vi "SetXAxisFormat.vi"(1 "Waveform Chart Reference":refnum<vi>) -> ()   [LabVIEW 2019]
uses:
  <vilib>/Utility/config.llb/Read Key (String).vi
  <vilib>/Utility/config.llb/NI_LVConfig.lvlib
panel:
  in  "Error In":errorcluster
  out "Error Out":errorcluster
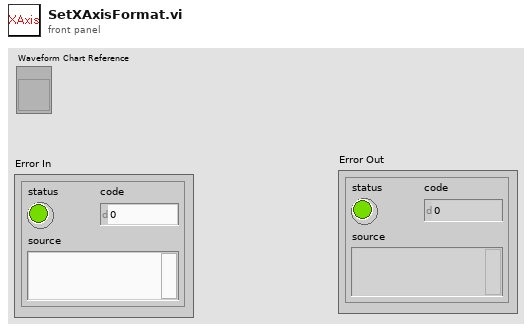
[diagram p1: front panel]
types:
  T1 = cluster{"XScale.Format":u8, "XScale.FormatString":string}[]
  T2 = typedef "NI_LVConfig.lvlib/Config Data RefNum.ctl" = refnum<k1>
  T3 = cluster{"XScale.Format":u8, "XScale.FormatString":string}
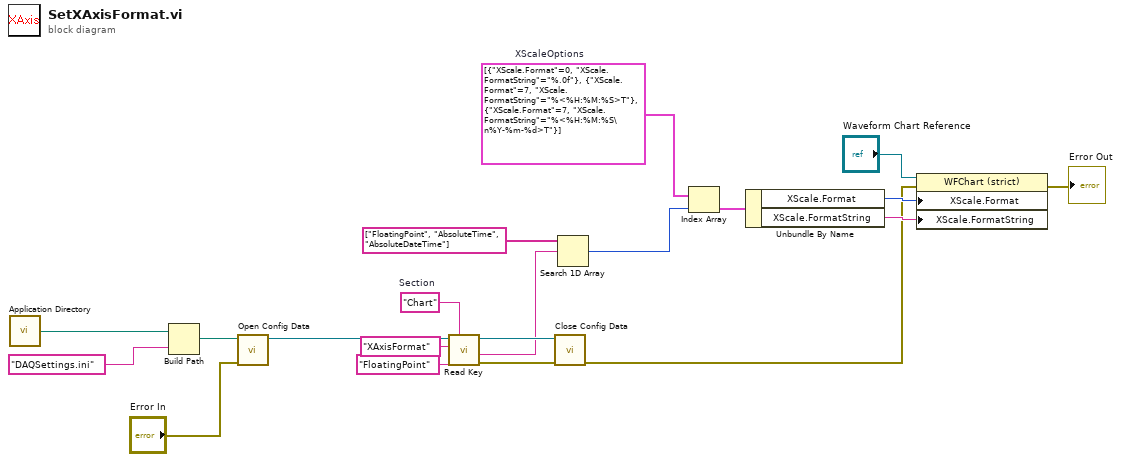
[diagram p0: block diagram]
diagram:
  w12 = "Chart"  # Section
  w4 = T1 [{"XScale.Format"=0, "XScale.FormatString"="%.0f"}, {"XScale.Format"=7, "XScale.FormatString"="%<%H:%M:%S>T"}, {"XScale.Format"=7, "XScale.FormatString"="%<%H:%M:%S\n%Y-%m-%d>T"}]  # XScaleOptions
  n1 = call <vilib>:"Application Directory.vi"() -> ("Application Directory"=w16:path)
  n2 = Build Path(base path=w16, name or relative path="DAQSettings.ini") -> (appended path=w14:path)
  n3 = call <vilib>:"Open Config Data.vi"("error in (no error)"="Error In", "configuration file path"=w14) -> ("refnum"=w9:T2)  [unwired: 7 in, 2 out]
  n4 = call-poly <vilib>:"Read Key.vi"("section"=w12, "default value"="FloatingPoint", "key"="XAxisFormat", "refnum"=w9) -> ("error out"=w10:errorcluster, "value"=w2:string, "refnum out"=w11:T2)  [unwired: 4 in, 1 out]
  n5 = call <vilib>:"Close Config Data.vi"("error in (no error)"=w10, "refnum"=w11) -> ("error out"=w6:errorcluster)  [unwired: 8 in, 1 out]
  n6 = Search 1D Array(1D array=string[] ["FloatingPoint", "AbsoluteTime", "AbsoluteDateTime"], element=w2) -> (index of element=w1:i32)  [unwired: 1 in]
  n7 = Index Array(array=w4, index=w1) -> (element=w20:T3)
  n8 = Unbundle By Name(w20) -> ("XScale.Format"=w18:u8, "XScale.FormatString"=w17:string)
  n9 = property class="WFChart (strict)"(reference="Waveform Chart Reference", error in=w6, "XScale.Format"=w18, "XScale.FormatString"=w17) -> (error out=→"Error Out":errorcluster)  [unwired: 1 out]
